vi "MotorGetNamedPosition.vi"(4 "Name":string, 5 "Motor":string, 9 "MotorData":T1[](array[typedef])) -> (0 "Position":i32, 3 "Ok?":bool)   [LabVIEW 2009]
uses:
  Controls/MotorData.ctl
  Controls/MotorNamedPosition.ctl
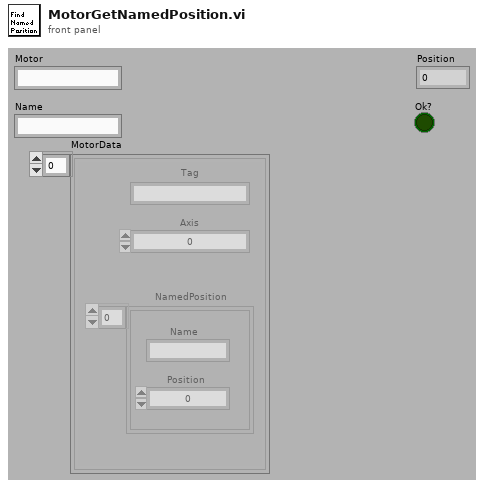
[diagram p1: front panel]
types:
  T1 = typedef "MotorData.ctl" = cluster{"Tag":string, "Axis":i32, "NamedPosition":T2[]}
  T2 = typedef "MotorNamedPosition.ctl" = cluster{"Position":i32, "Name":string}
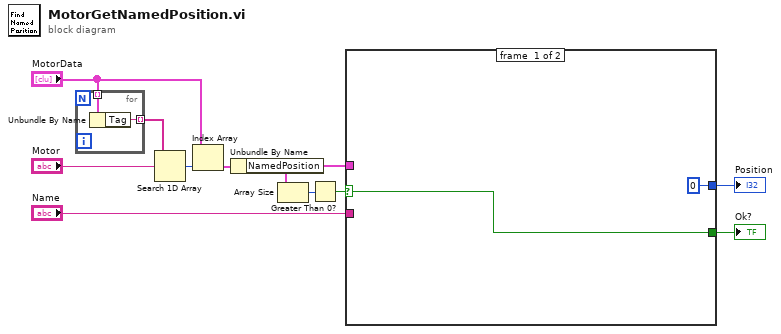
[diagram p0: block diagram]
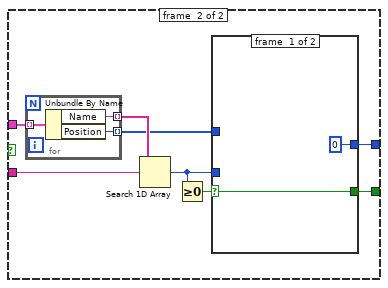
[diagram p2: hidden frame]
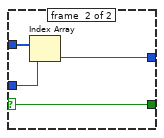
[diagram p3: hidden frame]
diagram:
  n1 = for {
    tunnel: [w13] -> w6 mode=indexing
    tunnel: "MotorData" -> [w12] mode=indexing
    n2 = Unbundle By Name(w12) -> ("Tag"=w13:string)
  }
  n3 = Search 1D Array(1D array=w6, element="Motor") -> (index of element=w9:i32)  [unwired: 1 out]
  n4 = Index Array(array="MotorData", index=w9) -> (element=w4:T1)
  n5 = Unbundle By Name(w4) -> ("NamedPosition"=w3:T2[])
  n6 = Array Size(array=w3) -> (size(s)=w2:i32)
  n7 = Greater Than 0?(x=w2) -> (x > 0?=w1:bool)
  n8 = case shown="True" w1 {
    selector: w1 -> [w15 _]
    tunnel: "Name" -> [_ w23]
    tunnel: [0 ("Position") w22] -> w8
    tunnel: [w15 w21] -> w7
    tunnel: w3 -> [_ w16]
    frame #0 {
    }
    frame #1 {
      n9 = for {
        tunnel: w16 -> [w32] mode=indexing
        tunnel: [w31] -> w20 mode=indexing
        tunnel: [w30] -> w19 mode=indexing
        n10 = Unbundle By Name(w32) -> ("Name"=w31:string, "Position"=w30:i32)
      }
      n11 = Search 1D Array(1D array=w20, element=w23) -> (index of element=w17:i32)  [unwired: 1 out]
      n12 = Greater Or Equal To 0?(x=w17) -> (x >= 0?=w18:bool)
      n13 = case shown="True" w18 {
        selector: w18 -> [w25 w26]
        tunnel: w19 -> [_ w29]
        tunnel: w17 -> [_ w28]
        tunnel: [0 ("Position") w27] -> w22
        tunnel: [w25 w26] -> w21
        frame #0 {
        }
        frame #1 {
          n14 = Index Array(array=w29, index=w28) -> (element=w27:i32)
        }
      }
    }
  }
  "Position" <- w8
  "Ok?" <- w7
